vi "Brake Pedal Released.vi"(8 "error in (no error)":errorcluster, 11 "Vehicle in":refnum<class "Vehicle.lvclass">) -> (0 "error out":errorcluster, 1 "Report Text":string, 2 "Test Result":bool, 3 "Vehicle out":refnum<class "Vehicle.lvclass">)   [LabVIEW 2024, in "Vehicle.lvclass"]
uses:
  Vehicle.lvclass
  Vehicle.lvclass/Vehicle.ctl
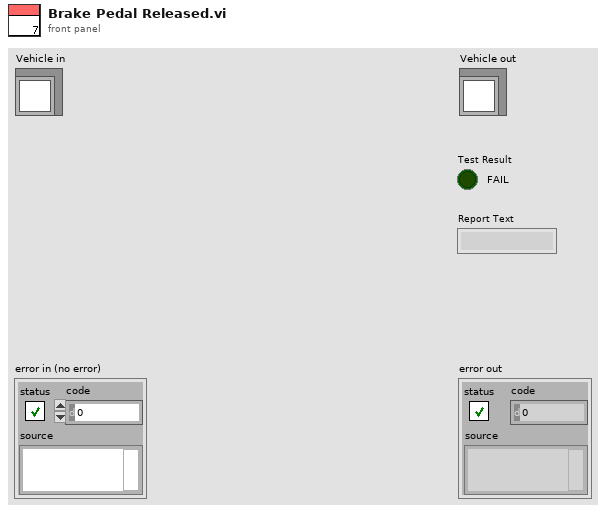
[diagram p1: front panel]
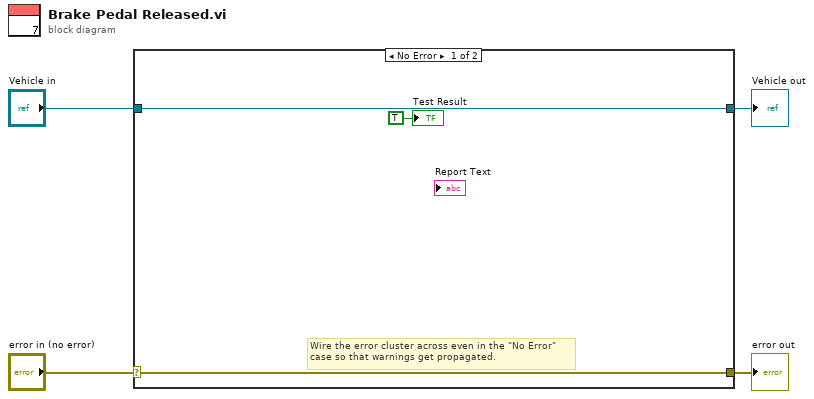
[diagram p0: block diagram]
diagram:
  n1 = case shown="No Error" "error in (no error)" {
    selector: "error in (no error)" -> [w6 w9]
    tunnel: [w6 w9] -> w3
    tunnel: [w7 w8] -> w1
    tunnel: "Vehicle in" -> [w7 w8]
    frame No Error {
      # "Wire the error cluster across even in the \"No Error\"\ncase so that warnings get propagated."
      "Test Result" <- TRUE ("Test Result")
    }
    frame Error {
    }
  }
  "error out" <- w3
  "Vehicle out" <- w1
